vi "Get SMO Port.vi"(8 "error in (no error)":errorcluster, 11 "RP100 in":refnum<class "RP100.lvclass">) -> (0 "error out":errorcluster, 2 "Port":u16, 3 "RP100 out":refnum<class "RP100.lvclass">)   [LabVIEW 2016, in "RP100.lvclass"]
uses:
  RP100.lvclass
  <userlib>/LevyLab/Levylab Instruments/Instrument Types/Strain/Instrument.Strain.lvclass
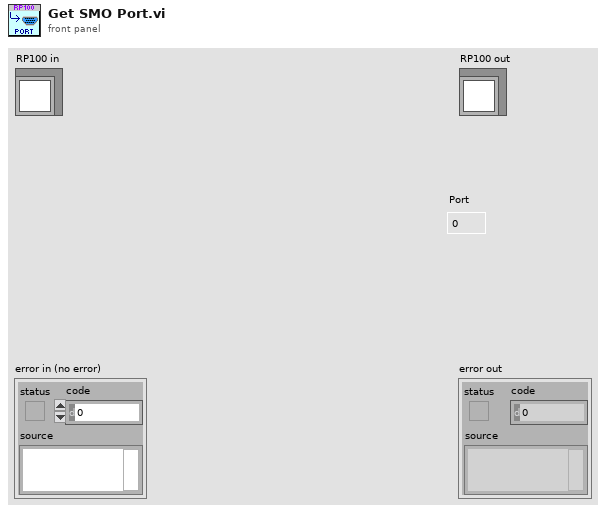
[diagram p1: front panel]
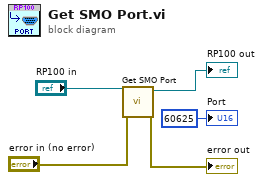
[diagram p0: block diagram]
diagram:
  n1 = call-parent "Get SMO Port.vi"("error in (no error)"="error in (no error)", "Instrument in"="RP100 in") -> ("error out"=→"error out":errorcluster, "Instrument out"=→"RP100 out":refnum<class "RP100.lvclass">)  [unwired: 7 in, 1 out]
  "Port" <- u16 60625 ("Port")
